vi "New Reference Recieved.vi"(8 "error in (no error)":errorcluster, 9 "Name":string, 10 "VI Refnum":refnum<vi>, 11 "Server in":refnum<class "Server.lvclass">) -> (0 "error out":errorcluster, 3 "Server out":refnum<class "Server.lvclass">)   [LabVIEW 2015, in "Server.lvlib" / "Server.lvclass"]
uses:
  Server.lvclass
  Server.lvclass/Server.ctl
  SubPanel User Interface Messages/Add New UI Msg/Add New UI Msg.lvclass/Add New UI Msg.ctl
  <vilib>/ActorFramework/Message Enqueuer/Message Enqueuer.lvclass/Message Enqueuer.ctl
  <vilib>/ActorFramework/Message Enqueuer/Enqueue.vi
  <vilib>/ActorFramework/Message Priority Queue/Priority Enqueue.vi
  SubPanel User Interface Messages/Add New UI Msg/Add New UI Msg.lvclass
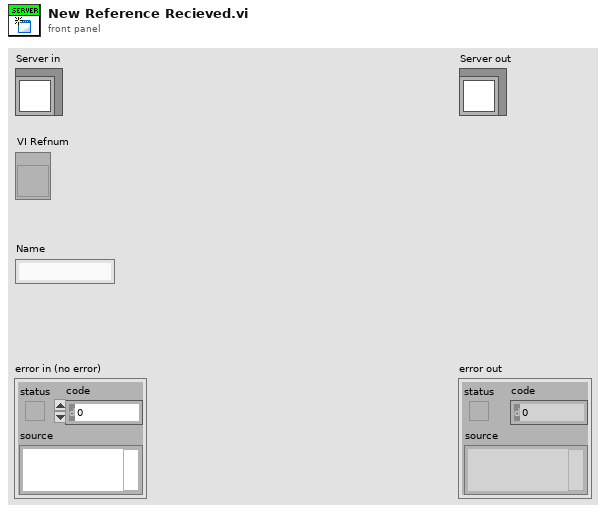
[diagram p1: front panel]
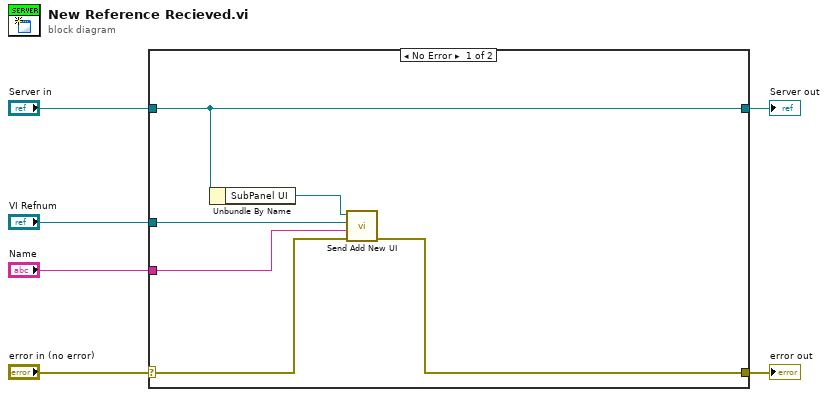
[diagram p0: block diagram]
diagram:
  n1 = case shown="No Error" "error in (no error)" {
    selector: "error in (no error)" -> [w9 w14]
    tunnel: [w8 w14] -> w5
    tunnel: [w12 w13] -> w3
    tunnel: "Server in" -> [w12 w13]
    tunnel: "VI Refnum" -> [w11 _]
    tunnel: "Name" -> [w10 _]
    frame No Error {
      n2 = Unbundle By Name(w12) -> ("SubPanel UI"=w7:refnum<class "Message Enqueuer.lvclass">)
      n3 = call "Send Add New UI.vi"("error in (no error)"=w9, "Name"=w10, "UI Reference"=w11, "Message Enqueuer"=w7) -> ("error out"=w8:errorcluster)  [unwired: 6 in, 1 out]
    }
    frame Error {
    }
  }
  "error out" <- w5
  "Server out" <- w3
